vi "Main.vi"() -> ()   [LabVIEW 2025]
panel:
  out "String":string
  in  "OK Button":bool
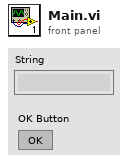
[diagram p1: front panel]
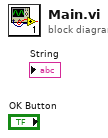
[diagram p0: block diagram]
diagram:
